vi "LabVIEW C Code Generation.vi"() -> ()   [LabVIEW 2023]
doc: "Demonstrates how to use the DFD FXP Code Generator VI to generate LabVIEW C code from a fixed-point filter.\n\nComplete the following steps to use this VI.\n1) Select a filter structure from <B>Target Structure</B>.\n2) Specify a <B>Destination Folder</B> for code generation.\n3) Specify a <B>Filter Name</B> for code generation.\n4) Run the VI.\n\n<B>Note:</B> Refer to the LabVIEW Help for information about restrictions on generating code from fixed-point filters."
uses:
  <vilib>/addons/Digital Filter Design/FXPModel.llb/DFD FXP Quantize Coef (Easy).vi
  <vilib>/addons/Digital Filter Design/CodeGen.llb/DFD FXP C Code Generator.vi
  <vilib>/addons/Digital Filter Design/NI_DigFilterLicensed.lvlib
panel:
  out "output files":path[](array[path])
  in  "Filter Name":string
  in  "Destination Folder":path
  out "Error Message":string
  in  "Target Structure":u16(ring)=1 items=["FIR Direct Form"=1, "FIR Direct Form Transposed"=2, "FIR Symmetric"=3, "FIR Antisymmetric"=4, "IIR Direct Form I"=5, "IIR Direct Form I Transposed"=6, "IIR Direct Form II"=7, "IIR Direct Form II Transposed"=8, "IIR Cascaded Second-Order Sections Form I"=9, "IIR Cascaded Second-Order Sections Form I Transposed"=10, "IIR Cascaded Second-Order Sections Form II"=11, "IIR Cascaded Second-Order Sections Form II Transposed"=12, "Lattice Allpass (basic sections)"=13, "Lattice Allpass (one multiplier sections)"=14, "Lattice Allpass (normalized sections)"=15, "Lattice AR (basic sections)"=16, "Lattice AR (one multiplier sections)"=17, "Lattice AR (normalized sections)"=18, "Lattice MA (minimum phase)"=19, "Lattice MA (maximum phase)"=20, "Lattice ARMA (basic sections)"=21, "Lattice ARMA (one multiplier sections)"=22, "Lattice ARMA (normalized sections)"=23]
  # "Select Help>>Show Context Help and move the cursor over the VI icon for more information."
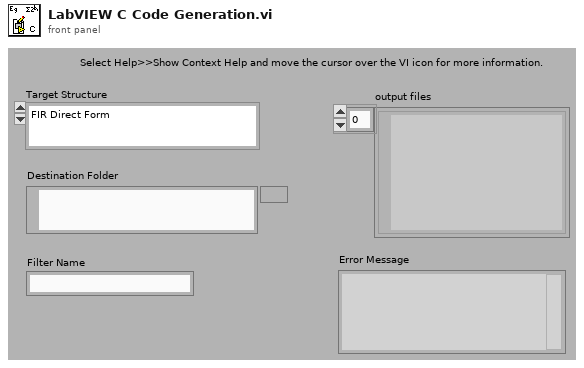
[diagram p1: front panel]
types:
  T1 = enum16{"Butterworth", "Chebyshev", "Inverse Chebyshev", "Elliptic", "Kaiser Window", "Dolph-Chebyshev Window", "Equi-Ripple FIR"}
  T2 = typedef "NI_DigFilterLicensed.lvlib/DFD Filter Obj.ctl" = cluster{"mSRate_Fs":dbl, "mSRate_Version":string, "mSRate_Comments":string, "mSRate_OrgCoef":T3, "mSRate_CurCoef":T3, "mSRate_Quantized?":bool, "mSRate_QCoef":T3, "mSRate_QSettings":T5[], "mSRate_Order":i32, "mSRate_Scaling":cluster{"mSRate_ScaleByPowerOf2?":bool, "mSRate_ScaleType":T7}}
  T3 = typedef "NI_DigFilterLicensed.lvlib/DFD Filter Coef.ctl" = cluster{"type":T4, "gain":dbl, "coef a (k)":dbl[], "coef b (v)":dbl[]}
  T4 = typedef "NI_DigFilterLicensed.lvlib/DFD Filter Structure Type Selector.ctl" = enum16{"Undefined", "FIR Direct Form", "FIR Direct Form Transposed", "FIR Symmetric", "FIR Antisymmetric", "IIR Direct Form I", "IIR Direct Form I Transposed", "IIR Direct Form II", "IIR Direct Form II Transposed", "IIR Cascaded Second Order Sections Form I", "IIR Cascaded Second Order Sections Form I Transposed", "IIR Cascaded Second Order Sections Form II", "IIR Cascaded Second Order Sections Form II Transposed", "Lattice Allpass (basic sections)", "Lattice Allpass (one multiplier sections)", "Lattice Allpass (normalized sections)", "Lattice AR (basic sections)", "Lattice AR (one multiplier sections)", "Lattice AR (normalized sections)", "Lattice MA (minimum phase)", "Lattice MA (maximum phase)", "Lattice ARMA (basic sections)", "Lattice ARMA (one multiplier sections)", "Lattice ARMA (normalized sections)"}
  T5 = typedef "NI_DigFilterLicensed.lvlib/dfd_Internal Quantization Settings.ctl" = cluster{"source":T6, "wl":i16, "iwl":i16, "overflow mode":enum16{"Saturation", "Wrap"}, "rounding mode":enum16{"Nearest", "Truncation"}, "signed?":bool}
  T6 = typedef "NI_DigFilterLicensed.lvlib/dfd_Internal Quantization Srcs.ctl" = u16
  T7 = typedef "NI_DigFilterLicensed.lvlib/DFD Coef Norm Type.ctl" = enum16{"No Norm", "Time Domain 1-Norm", "Time Domain 2-Norm", "Time Domain Inf-Norm"}
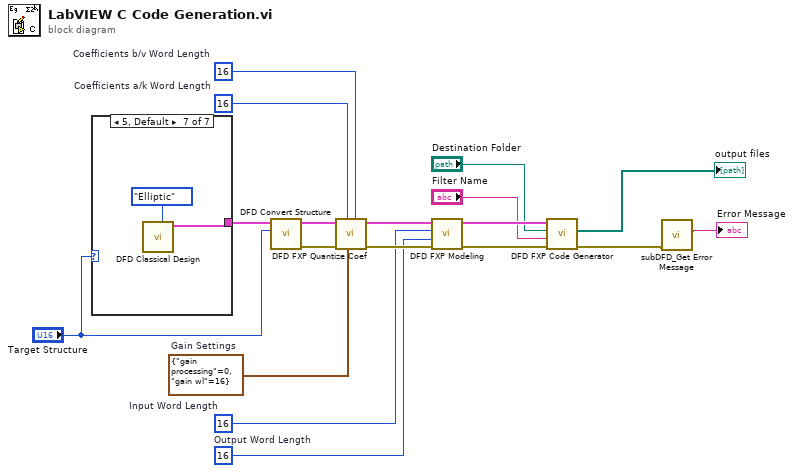
[diagram p0: block diagram]
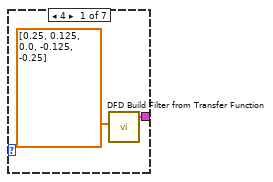
[diagram p2: hidden frame]
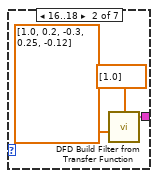
[diagram p3: hidden frame]
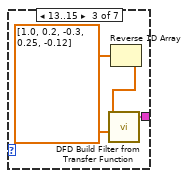
[diagram p4: hidden frame]
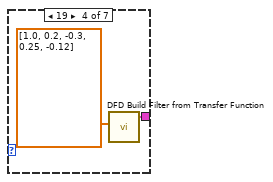
[diagram p5: hidden frame]
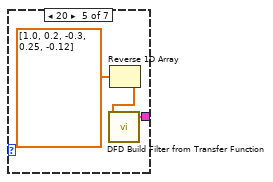
[diagram p6: hidden frame]
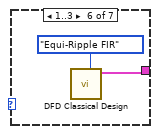
[diagram p7: hidden frame]
diagram:
  w8 = i16 16  # Output Word Length
  w9 = i16 16  # Input Word Length
  w12 = cluster{"gain processing":u16, "gain wl":i16} {"gain processing"=0, "gain wl"=16}  # Gain Settings
  w13 = i16 16  # Coefficients b/v Word Length
  w14 = i16 16  # Coefficients a/k Word Length
  n1 = case shown="5, Default" "Target Structure" {
    tunnel: [w20 w23 w26 w28 w31 w33 w35] -> w18
    frame 4 {
      n2 = call <vilib>:"DFD Build Filter from Transfer Function.vi"("numerator"=dbl[] [0.25, 0.125, 0.0, -0.125, -0.25]) -> ("filter out"=w20:T2)  [unwired: 3 in, 7 out]
    }
    frame 16..18 {
      n3 = call <vilib>:"DFD Build Filter from Transfer Function.vi"("denominator"=dbl[] [1.0, 0.2, -0.3, 0.25, -0.12] ("numerator"), "numerator"=dbl[] [1.0]) -> ("filter out"=w23:T2)  [unwired: 2 in, 7 out]
    }
    frame 13..15 {
      w25 = dbl[] [1.0, 0.2, -0.3, 0.25, -0.12] ("numerator")
      n4 = Reverse 1D Array(array=w25) -> (reversed array=w24:dbl[])
      n5 = call <vilib>:"DFD Build Filter from Transfer Function.vi"("denominator"=w25, "numerator"=w24) -> ("filter out"=w26:T2)  [unwired: 2 in, 7 out]
    }
    frame 19 {
      n6 = call <vilib>:"DFD Build Filter from Transfer Function.vi"("numerator"=dbl[] [1.0, 0.2, -0.3, 0.25, -0.12]) -> ("filter out"=w28:T2)  [unwired: 3 in, 7 out]
    }
    frame 20 {
      n7 = Reverse 1D Array(array=dbl[] [1.0, 0.2, -0.3, 0.25, -0.12] ("numerator")) -> (reversed array=w29:dbl[])
      n8 = call <vilib>:"DFD Build Filter from Transfer Function.vi"("numerator"=w29) -> ("filter out"=w31:T2)  [unwired: 3 in, 7 out]
    }
    frame 1..3 {
      n9 = call <vilib>:"DFD Classical Design.vi"("design method"=T1."Equi-Ripple FIR") -> ("filter out"=w33:T2)  [unwired: 5 in, 5 out]
    }
    frame 5, Default {
      n10 = call <vilib>:"DFD Classical Design.vi"("design method"=T1."Elliptic") -> ("filter out"=w35:T2)  [unwired: 5 in, 5 out]
    }
  }
  n11 = call <vilib>:"DFD Convert Structure.vi"("target structure"="Target Structure", "filter in"=w18) -> ("error out"=w15:errorcluster, "filter out"=w16:T2)  [unwired: 1 in, 7 out]
  n12 = call-poly <vilib>:"DFD FXP Quantize Coef.vi"("coefficients b/v word length"=w13, "gain settings"=w12, "coefficients a/k word length"=w14, "error in (no error)"=w15, "filter in"=w16) -> ("error out"=w10:errorcluster, "filter out"=w11:T2)  [unwired: 5 out]
  n13 = call <vilib>:"DFD FXP Modeling.vi"("error in (no error)"=w10, "output word length"=w8, "input word length"=w9, "filter in"=w11) -> ("error out"=w6:errorcluster, "filter out"=w7:T2)  [unwired: 3 in, 3 out]
  n14 = call-poly <vilib>:"DFD FXP Code Generator.vi"("error in (no error)"=w6, "filter name"="Filter Name", "destination folder"="Destination Folder", "filter in"=w7) -> ("error out"=w2:errorcluster, "output files"=→"output files":path[])  [unwired: 3 in, 3 out]
  n15 = call <vilib>:"subDFD_Get Error Message.vi"("error in (no error)"=w2) -> ("Error Message"=→"Error Message":string)  [unwired: 10 out]
